vi "test_read-nmea-data2.vi"() -> ()   [LabVIEW 2019] (continued)
1.05,4*0A\n\t\n15:09:20.38\tF9P\t$GPGSV,3,1,09,02,54,318,23,04,19,044,21,05,36,246,28,06,65,046,30,1*66\n\t\n15:09:20.40\tF9P\t$GPGSV,3,2,09,09,45,075,25,12,24,278,29,17,34,153,23,19,53,156,23,1*68\n\t\n15:09:20.42\tF9P\t$GPGSV,3,3,09,25,12,308,,1*52\n\t\n15:09:20.44\tF9P\t$GPGSV,3,1,09,02,54,318,,04,19,044,15,05,36,246,18,06,65,046,22,6*67\n\t\n15:09:20.46\tF9P\t$GPGSV,3,2,09,09,45,075,18,12,24,278,17,17,34,153,,19,53,156,,6*6C\n\t\n15:09:20.48\tF9P\t$GPGSV,3,3,09,25,12,308,,6*55\n\t\n15:09:20.50\tF9P\t$GLGSV,2,1,08,69,13,031,,70,73,042,,71,50,204,32,72,03,209,,1*70\n\t\n15:09:20.52\tF9P\t$GLGSV,2,2,08,77,01,327,,84,21,121,13,85,70,063,25,86,35,329,,1*70\n\t\n15:09:20.54\tF9P\t$GLGSV,2,1,08,69,13,031,17,70,73,042,,71,50,204,23,72,03,209,,3*74\n\t\n15:09:20.56\tF9P\t$GLGSV,2,2,08,77,01,327,,84,21,121,17,85,70,063,20,86,35,329,,3*73\n\t\n15:09:20.58\tF9P\t$GAGSV,2,1,08,02,09,298,11,04,65,120,30,09,30,193,18,11,70,356,20,7*7A\n\t\n15:09:20.60\tF9P\t$GAGSV,2,2,08,12,41,101,18,19,27,046,08,25,10,250,,36,25,307,18,7*7D\n\t\n15:09:20.62\tF9P\t$GAGSV,2,1,08,02,09,298,,04,65,120,32,09,30,193,17,11,70,356,18,2*79\n\t\n15:09:20.64\tF9P\t$GAGSV,2,2,08,12,41,101,17,19,27,046,,25,10,250,,36,25,307,22,2*76\n\t\n15:09:20.66\tF9P\t$GBGSV,1,1,03,11,51,130,21,14,86,148,25,33,59,218,25,1*41\n\t\n15:09:20.68\tF9P\t$GBGSV,1,1,04,08,,,24,11,51,130,20,14,86,148,25,33,59,218,,3*4C\n\t\n15:09:20.70\tF9P\t$GNGLL,3723.60443,N,12656.90761,E,060922.00,A,A*77\n\t\n15:09:20.72\tF9P\t\t\n15:09:20.74\tF9P\t\t\n15:09:20.76\tF9P\t\t\n15:09:20.78\tF9P\t\t\n15:09:20.80\tF9P\t\t\n15:09:20.82\tF9P\t\t\n15:09:20.84\tF9P\t\t\n15:09:20.86\tF9P\t\t\n15:09:20.88\tF9P\t\t\n15:09:20.90\tF9P\t\t\n15:09:20.92\tF9P\t\t\n15:09:20.94\tF9P\t\t\n15:09:20.96\tF9P\t\t\n15:09:20.98\tF9P\t\t\n15:09:21.00\tF9P\t\t\n15:09:21.02\tF9P\t\t\n15:09:21.04\tF9P\t\t\n15:09:21.06\tF9P\t\t\n15:09:21.08\tF9P\t\t\n15:09:21.10\tF9P\t\t\n15:09:21.12\tF9P\t\t\n15:09:21.14\tF9P\t\t\n15:09:21.16\tF9P\t\t\n15:09:21.18\tF9P\t\t\n15:09:21.20\tF9P\t\t\n15:09:21.22\tF9P\t\t\n15:09:21.24\tF9P\t$GNRMC,060923.00,A,3723.60417,N,12656.90709,E,1.682,,250720,,,A,V*15\n\t\n15:09:21.26\tF9P\t$GNVTG,,T,,M,1.682,N,3.115,K,A*36\n\t\n15:09:21.28\tF9P\t$GNGGA,060923.00,3723.60417,N,12656.90709,E,1,12,0.73,58.2,M,18.5,M,,*78\n\t\n15:09:21.30\tF9P\t$GNGSA,A,3,12,06,19,05,17,09,04,02,,,,,1.28,0.73,1.05,1*0B\n\t\n15:09:21.32\tF9P\t$GNGSA,A,3,85,71,84,,,,,,,,,,1.28,0.73,1.05,2*0E\n\t\n15:09:21.34\tF9P\t$GNGSA,A,3,36,19,11,04,09,12,,,,,,,1.28,0.73,1.05,3*0B\n\t\n15:09:21.36\tF9P\t$GNGSA,A,3,14,11,33,,,,,,,,,,1.28,0.73,1.05,4*0A\n\t\n15:09:21.38\tF9P\t$GPGSV,3,1,09,02,54,318,24,04,19,044,20,05,36,246,28,06,65,046,30,1*60\n\t\n15:09:21.40\tF9P\t$GPGSV,3,2,09,09,45,075,25,12,24,278,29,17,34,153,23,19,53,156,24,1*6F\n\t\n15:09:21.42\tF9P\t$GPGSV,3,3,09,25,12,308,,1*52\n\t\n15:09:21.44\tF9P\t$GPGSV,3,1,09,02,54,318,,04,19,044,14,05,36,246,18,06,65,046,24,6*60\n\t\n15:09:21.46\tF9P\t$GPGSV,3,2,09,09,45,075,18,12,24,278,18,17,34,153,,19,53,156,,6*63\n\t\n15:09:21.48\tF9P\t$GPGSV,3,3,09,25,12,308,,6*55\n\t\n15:09:21.50\tF9P\t$GLGSV,2,1,08,69,13,031,,70,73,042,,71,50,204,28,72,03,209,,1*7B\n\t\n15:09:21.52\tF9P\t$GLGSV,2,2,08,77,01,327,,84,21,121,11,85,70,063,30,86,35,329,,1*76\n\t\n15:09:21.54\tF9P\t$GLGSV,2,1,08,69,13,031,19,70,73,042,,71,50,204,22,72,03,209,,3*7B\n\t\n15:09:21.56\tF9P\t$GLGSV,2,2,08,77,01,327,,84,21,121,19,85,70,063,20,86,35,329,,3*7D\n\t\n15:09:21.58\tF9P\t$GAGSV,2,1,08,02,09,298,15,04,65,120,21,09,30,193,17,11,70,356,20,7*71\n\t\n15:09:21.60\tF9P\t$GAGSV,2,2,08,12,41,101,20,19,27,046,17,25,10,250,,36,25,307,20,7*73\n\t\n15:09:21.62\tF9P\t$GAGSV,2,1,08,02,09,298,,04,65,120,27,09,30,193,17,11,70,356,18,2*7D\n\t\n15:09:21.64\tF9P\t$GAGSV,2,2,08,12,41,101,16,19,27,046,,25,10,250,,36,25,307,19,2*7F\n\t\n15:09:21.66\tF9P\t$GBGSV,1,1,03,11,51,130,22,14,86,148,25,33,59,218,26,1*41\n\t\n15:09:21.68\tF9P\t$GBGSV,1,1,04,08,,,25,11,51,130,21,14,86,148,24,33,59,218,,3*4D\n\t\n15:09:21.70\tF9P\t$GNGLL,3723.60417,N,12656.90709,E,060923.00,A,A*79\n\t\n15:09:21.72\tF9P\t\t\n15:09:21.74\tF9P\t\t\n15:09:21.76\tF9P\t\t\n15:09:21.78\tF9P\t\t\n15:09:21.80\tF9P\t\t\n15:09:21.82\tF9P\t\t\n15:09:21.84\tF9P\t\t\n15:09:21.86\tF9P\t\t\n15:09:21.88\tF9P\t\t\n15:09:21.90\tF9P\t\t\n15:09:21.92\tF9P\t\t\n15:09:21.94\tF9P\t\t\n15:09:21.96\tF9P\t\t\n15:09:21.98\tF9P\t\t\n15:09:22.00\tF9P\t\t\n15:09:22.02\tF9P\t\t\n15:09:22.04\tF9P\t\t\n15:09:22.06\tF9P\t\t\n15:09:22.08\tF9P\t\t\n15:09:22.10\tF9P\t\t\n15:09:22.12\tF9P\t\t\n15:09:22.14\tF9P\t\t\n15:09:22.16\tF9P\t\t\n15:09:22.18\tF9P\t\t\n15:09:22.20\tF9P\t\t\n15:09:22.22\tF9P\t\t\n15:09:22.24\tF9P\t$GNRMC,060924.00,A,3723.60402,N,12656.90651,E,1.519,,250720,,,A,V*1B\n\t\n15:09:22.26\tF9P\t$GNVTG,,T,,M,1.519,N,2.813,K,A*39\n\t\n15:09:22.28\tF9P\t$GNGGA,060924.00,3723.60402,N,12656.90651,E,1,12,0.73,58.0,M,18.5,M,,*75\n\t\n15:09:22.30\tF9P\t$GNGSA,A,3,12,06,19,05,17,09,04,02,,,,,1.28,0.73,1.05,1*0B\n\t\n15:09:22.32\tF9P\t$GNGSA,A,3,85,71,84,,,,,,,,,,1.28,0.73,1.05,2*0E\n\t\n15:09:22.34\tF9P\t$GNGSA,A,3,36,19,11,04,09,12,,,,,,,1.28,0.73,1.05,3*0B\n\t\n15:09:22.36\tF9P\t$GNGSA,A,3,14,11,33,,,,,,,,,,1.28,0.73,1.05,4*0A\n\t\n15:09:22.38\tF9P\t$GPGSV,3,1,09,02,54,318,23,04,19,044,19,05,36,246,28,06,65,046,28,1*64\n\t\n15:09:22.40\tF9P\t$GPGSV,3,2,09,09,45,075,25,12,24,278,29,17,34,153,25,19,53,156,24,1*69\n\t\n15:09:22.43\tF9P\t$GPGSV,3,3,09,25,12,307,,1*5D\n\t\n15:09:22.45\tF9P\t$GPGSV,3,1,09,02,54,318,,04,19,044,13,05,36,246,20,06,65,046,23,6*6B\n\t\n15:09:22.47\tF9P\t$GPGSV,3,2,09,09,45,075,18,12,24,278,16,17,34,153,,19,53,156,,6*6D\n\t\n15:09:22.49\tF9P\t$GPGSV,3,3,09,25,12,307,,6*5A\n\t\n15:09:22.51\tF9P\t$GLGSV,2,1,08,69,13,031,,70,73,042,,71,50,204,28,72,03,209,,1*7B\n\t\n15:09:22.53\tF9P\t$GLGSV,2,2,08,77,01,327,,84,21,121,10,85,70,063,25,86,35,329,,1*73\n\t\n15:09:22.55\tF9P\t$GLGSV,2,1,08,69,13,031,20,70,73,042,,71,50,204,22,72,03,209,,3*71\n\t\n15:09:22.57\tF9P\t$GLGSV,2,2,08,77,01,327,,84,21,121,18,85,70,063,21,86,35,329,,3*7D\n\t\n15:09:22.59\tF9P\t$GAGSV,2,1,08,02,09,298,23,04,65,120,21,09,30,193,16,11,70,356,19,7*7F\n\t\n15:09:22.61\tF9P\t$GAGSV,2,2,08,12,41,101,19,19,27,046,10,25,10,250,,36,25,307,21,7*7F\n\t\n15:09:22.63\tF9P\t$GAGSV,2,1,08,02,09,298,,04,65,120,33,09,30,193,14,11,70,356,16,2*75\n\t\n15:09:22.65\tF9P\t$GAGSV,2,2,08,12,41,101,13,19,27,046,,25,10,250,,36,25,307,18,2*7B\n\t\n15:09:22.67\tF9P\t$GBGSV,1,1,03,11,51,130,22,14,86,148,26,33,59,218,25,1*41\n\t\n15:09:22.69\tF9P\t$GBGSV,1,1,04,08,,,24,11,51,130,21,14,86,148,25,33,59,218,,3*4D\n\t\n15:09:22.71\tF9P\t$GNGLL,3723.60402,N,12656.90651,E,060924.00,A,A*76\n\t\n15:09:22.73\tF9P\t\t\n15:09:22.75\tF9P\t\t\n15:09:22.77\tF9P\t\t\n15:09:22.79\tF9P\t\t\n15:09:22.81\tF9P\t\t\n15:09:22.83\tF9P\t\t\n15:09:22.85\tF9P\t\t\n15:09:22.87\tF9P\t\t\n15:09:22.89\tF9P\t\t\n15:09:22.91\tF9P\t\t\n15:09:22.93\tF9P\t\t\n15:09:22.95\tF9P\t\t\n15:09:22.97\tF9P\t\t\n15:09:22.99\tF9P\t\t\n15:09:23.01\tF9P\t\t\n15:09:23.03\tF9P\t\t\n15:09:23.05\tF9P\t\t\n15:09:23.07\tF9P\t\t\n15:09:23.09\tF9P\t\t\n15:09:23.11\tF9P\t\t\n15:09:23.13\tF9P\t\t\n15:09:23.15\tF9P\t\t\n15:09:23.17\tF9P\t\t\n15:09:23.19\tF9P\t\t\n15:09:23.21\tF9P\t\t\n15:09:23.23\tF9P\t\t\n15:09:23.25\tF9P\t$GNRMC,060925.00,A,3723.60390,N,12656.90580,E,1.871,,250720,,,A,V*1A\n\t\n15:09:23.27\tF9P\t$GNVTG,,T,,M,1.871,N,3.465,K,A*36\n\t\n15:09:23.29\tF9P\t$GNGGA,060925.00,3723.60390,N,12656.90580,E,1,12,0.76,57.8,M,18.5,M,,*75\n\t\n15:09:23.32\tF9P\t$GNGSA,A,3,12,06,19,05,17,09,04,02,,,,,1.33,0.76,1.09,1*08\n\t\n15:09:23.34\tF9P\t$GNGSA,A,3,85,71,84,,,,,,,,,,1.33,0.76,1.09,2*0D\n\t\n15:09:23.36\tF9P\t$GNGSA,A,3,36,19,11,04,09,12,,,,,,,1.33,0.76,1.09,3*08\n\t\n15:09:23.38\tF9P\t$GNGSA,A,3,14,11,33,,,,,,,,,,1.33,0.76,1.09,4*09\n\t\n15:09:23.40\tF9P\t$GPGSV,3,1,09,02,54,318,24,04,19,044,20,05,36,246,29,06,65,046,28,1*68\n\t\n15:09:23.42\tF9P\t$GPGSV,3,2,09,09,45,075,24,12,24,278,28,17,34,153,23,19,53,156,23,1*68\n\t\n15:09:23.44\tF9P\t$GPGSV,3,3,09,25,12,307,26,1*59\n\t\n15:09:23.46\tF9P\t$GPGSV,3,1,09,02,54,318,,04,19,044,13,05,36,246,20,06,65,046,20,6*68\n\t\n15:09:23.48\tF9P\t$GPGSV,3,2,09,09,45,075,19,12,24,278,16,17,34,153,,19,53,156,,6*6C\n\t\n15:09:23.50\tF9P\t$GPGSV,3,3,09,25,12,307,,6*5A\n\t\n15:09:23.52\tF9P\t$GLGSV,2,1,08,69,13,031,,70,73,042,,71,50,204,27,72,03,209,,1*74\n\t\n15:09:23.54\tF9P\t$GLGSV,2,2,08,77,01,327,,84,21,121,07,85,70,063,25,86,35,329,,1*75\n\t\n15:09:23.56\tF9P\t$GLGSV,2,1,08,69,13,031,22,70,73,042,,71,50,204,23,72,03,209,,3*72\n\t\n15:09:23.58\tF9P\t$GLGSV,2,2,08,77,01,327,,84,21,121,18,85,70,063,22,86,35,329,,3*7E\n\t\n15:09:23.60\tF9P\t$GAGSV,2,1,08,02,09,298,22,04,65,120,23,09,30,193,16,11,70,356,20,7*76\n\t\n15:09:23.62\tF9P\t$GAGSV,2,2,08,12,41,101,19,19,27,046,13,25,10,250,,36,25,307,22,7*7F\n\t\n15:09:23.64\tF9P\t$GAGSV,2,1,08,02,09,298,,04,65,120,32,09,30,193,13,11,70,356,19,2*7C\n\t\n15:09:23.66\tF9P\t$GAGSV,2,2,08,12,41,101,,19,27,046,,25,10,250,,36,25,307,16,2*77\n\t\n15:09:23.68\tF9P\t$GBGSV,1,1,03,11,51,130,22,14,86,148,26,33,59,218,30,1*45\n\t\n15:09:23.70\tF9P\t$GBGSV,1,1,04,08,,,23,11,51,130,23,14,86,148,26,33,59,218,,3*4B\n\t\n15:09:23.72\tF9P\t$GNGLL,3723.60390,N,12656.90580,E,060925.00,A,A*74\n\t\n15:09:23.74\tF9P\t\t\n15:09:23.76\tF9P\t\t\n15:09:23.78\tF9P\t\t\n15:09:23.80\tF9P\t\t\n15:09:23.82\tF9P\t\t\n15:09:23.84\tF9P\t\t\n15:09:23.86\tF9P\t\t\n15:09:23.88\tF9P\t\t\n15:09:23.90\tF9P\t\t\n15:09:23.92\tF9P\t\t\n15:09:23.94\tF9P\t\t\n15:09:23.96\tF9P\t\t\n15:09:23.98\tF9P\t\t\n15:09:24.00\tF9P\t\t\n15:09:24.02\tF9P\t\t\n15:09:24.04\tF9P\t\t\n15:09:24.06\tF9P\t\t\n15:09:24.08\tF9P\t\t\n15:09:24.10\tF9P\t\t\n15:09:24.12\tF9P\t\t\n15:09:24.14\tF9P\t\t\n15:09:24.16\tF9P\t\t\n15:09:24.18\tF9P\t\t\n15:09:24.20\tF9P\t\t\n15:09:24.22\tF9P\t\t\n15:09:24.24\tF9P\t$GNRMC,060926.00,A,3723.60386,N,12656.90524,E,1.422,,250720,,,A,V*1A\n\t\n15:09:24.26\tF9P\t$GNVTG,,T,,M,1.422,N,2.634,K,A*3B\n\t\n15:09:24.28\tF9P\t$GNGGA,060926.00,3723.60386,N,12656.90524,E,1,12,0.66,58.2,M,18.5,M,,*7B\n\t\n15:09:24.30\tF9P\t$GNGSA,A,3,12,06,19,05,17,09,04,02,,,,,1.21,0.66,1.01,1*02\n\t\n15:09:24.32\tF9P\t$GNGSA,A,3,85,71,84,,,,,,,,,,1.21,0.66,1.01,2*07\n\t\n15:09:24.34\tF9P\t$GNGSA,A,3,36,19,11,04,09,12,,,,,,,1.21,0.66,1.01,3*02\n\t\n15:09:24.36\tF9P\t$GNGSA,A,3,14,11,33,,,,,,,,,,1.21,0.66,1.01,4*03\n\t\n15:09:24.38\tF9P\t$GPGSV,3,1,09,02,54,318,24,04,19,044,20,05,36,246,27,06,65,046,29,1*67\n\t\n15:09:24.40\tF9P\t$GPGSV,3,2,09,09,45,075,25,12,24,278,27,17,34,153,23,19,53,156,23,1*66\n\t\n15:09:24.42\tF9P\t$GPGSV,3,3,09,25,12,307,31,1*5F\n\t\n15:09:24.44\tF9P\t$GPGSV,3,1,09,02,54,318,,04,19,044,14,05,36,246,20,06,65,046,18,6*64\n\t\n15:09:24.46\tF9P\t$GPGSV,3,2,09,09,45,075,20,12,24,278,15,17,34,153,,19,53,156,,6*65\n\t\n15:09:24.48\tF9P\t$GPGSV,3,3,09,25,12,307,,6*5A\n\t\n15:09:24.50\tF9P\t$GLGSV,2,1,08,69,13,031,,70,73,042,,71,50,204,25,72,03,209,,1*76\n\t\n15:09:24.52\tF9P\t$GLGSV,2,2,08,77,01,327,,84,21,121,13,85,70,063,26,86,35,329,,1*73\n\t\n15:09:24.54\tF9P\t$GLGSV,2,1,08,69,13,031,21,70,73,042,,71,50,204,22,72,03,209,,3*70\n\t\n15:09:24.56\tF9P\t$GLGSV,2,2,08,77,01,327,,84,21,121,16,85,70,063,22,86,35,329,,3*70\n\t\n15:09:24.58\tF9P\t$GAGSV,2,1,08,02,09,298,26,04,65,120,26,09,30,193,15,11,70,356,20,7*74\n\t\n15:09:24.60\tF9P\t$GAGSV,2,2,08,12,41,101,19,19,27,046,13,25,10,250,,36,25,307,34,7*78\n\t\n15:09:24.62\tF9P\t$GAGSV,2,1,08,02,09,298,,04,65,120,35,09,30,193,11,11,70,356,19,2*79\n\t\n15:09:24.64\tF9P\t$GAGSV,2,2,08,12,41,101,,19,27,046,,25,10,250,,36,25,307,,2*70\n\t\n15:09:24.66\tF9P\t$GBGSV,1,1,03,11,51,130,23,14,86,148,26,33,59,218,24,1*41\n\t\n15:09:24.68\tF9P\t$GBGSV,1,1,04,08,,,23,11,51,130,23,14,86,148,26,33,59,218,,3*4B\n\t\n15:09:24.70\tF9P\t$GNGLL,3723.60386,N,12656.90524,E,060926.00,A,A*7E\n\t\n15:09:24.72\tF9P\t\t\n15:09:24.74\tF9P\t\t\n15:09:24.76\tF9P\t\t\n15:09:24.78\tF9P\t\t\n15:09:24.80\tF9P\t\t\n15:09:24.82\tF9P\t\t\n15:09:24.84\tF9P\t\t\n15:09:24.86\tF9P\t\t\n15:09:24.88\tF9P\t\t\n15:09:24.90\tF9P\t\t\n15:09:24.92\tF9P\t\t\n15:09:24.94\tF9P\t\t\n15:09:24.96\tF9P\t\t\n15:09:24.98\tF9P\t\t\n15:09:25.00\tF9P\t\t\n15:09:25.02\tF9P\t\t\n15:09:25.04\tF9P\t\t\n15:09:25.06\tF9P\t\t\n15:09:25.08\tF9P\t\t\n15:09:25.10\tF9P\t\t\n15:09:25.12\tF9P\t\t\n15:09:25.14\tF9P\t\t\n15:09:25.16\tF9P\t\t\n15:09:25.18\tF9P\t\t\n15:09:25.20\tF9P\t\t\n15:09:25.22\tF9P\t\t\n15:09:25.24\tF9P\t$GNRMC,060927.00,A,3723.60381,N,12656.90446,E,2.414,257.19,250720,,,A,V*09\n\t\n15:09:25.26\tF9P\t$GNVTG,257.19,T,,M,2.414,N,4.470,K,A*2F\n\t\n15:09:25.28\tF9P\t$GNGGA,060927.00,3723.60381,N,12656.90446,E,1,12,0.66,57.8,M,18.5,M,,*7D\n\t\n15:09:25.30\tF9P\t$GNGSA,A,3,12,06,19,05,17,09,04,02,,,,,1.21,0.66,1.01,1*02\n\t\n15:09:25.32\tF9P\t$GNGSA,A,3,85,71,84,,,,,,,,,,1.21,0.66,1.01,2*07\n\t\n15:09:25.34\tF9P\t$GNGSA,A,3,36,19,11,04,09,12,,,,,,,1.21,0.66,1.01,3*02\n\t\n15:09:25.36\tF9P\t$GNGSA,A,3,14,11,33,,,,,,,,,,1.21,0.66,1.01,4*03\n\t\n15:09:25.38\tF9P\t$GPGSV,3,1,09,02,54,318,24,04,19,044,19,05,36,246,27,06,65,046,34,1*61\n\t\n15:09:25.40\tF9P\t$GPGSV,3,2,09,09,45,075,27,12,24,278,26,17,34,153,21,19,53,156,22,1*66\n\t\n15:09:25.42\tF9P\t$GPGSV,3,3,09,25,12,307,31,1*5F\n\t\n15:09:25.44\tF9P\t$GPGSV,3,1,09,02,54,318,,04,19,044,13,05,36,246,21,06,65,046,20,6*69\n\t\n15:09:25.46\tF9P\t$GPGSV,3,2,09,09,45,075,19,12,24,278,16,17,34,153,,19,53,156,,6*6C\n\t\n15:09:25.48\tF9P\t$GPGSV,3,3,09,25,12,307,,6*5A\n\t\n15:09:25.50\tF9P\t$GLGSV,2,1,08,69,13,031,,70,73,042,,71,50,204,25,72,03,209,,1*76\n\t\n15:09:25.52\tF9P\t$GLGSV,2,2,08,77,01,327,,84,21,121,13,85,70,063,25,86,35,329,,1*70\n\t\n15:09:25.54\tF9P\t$GLGSV,2,1,08,69,13,031,21,70,73,042,,71,50,204,21,72,03,209,,3*73\n\t\n15:09:25.56\tF9P\t$GLGSV,2,2,08,77,01,327,,84,21,121,15,85,70,063,21,86,35,329,,3*70\n\t\n15:09:25.58\tF9P\t$GAGSV,2,1,08,02,09,298,25,04,65,120,24,09,30,193,15,11,70,356,19,7*7F\n\t\n15:09:25.60\tF9P\t$GAGSV,2,2,08,12,41,101,18,19,27,046,14,25,10,250,,36,25,307,32,7*78\n\t\n15:09:25.62\tF9P\t$GAGSV,2,1,08,02,09,298,,04,65,120,26,09,30,193,,11,70,356,20,2*71\n\t\n15:09:25.64\tF9P\t$GAGSV,2,2,08,12,41,101,,19,27,046,,25,10,250,,36,25,307,,2*70\n\t\n15:09:25.66\tF9P\t$GBGSV,1,1,03,11,51,130,22,14,86,148,25,33,59,218,29,1*4E\n\t\n15:09:25.68\tF9P\t$GBGSV,1,1,04,08,,,22,11,51,130,23,14,86,148,30,33,59,218,,3*4D\n\t\n15:09:25.70\tF9P\t$GNGLL,3723.60381,N,12656.90446,E,060927.00,A,A*7D\n\t\n15:09:25.72\tF9P\t\t\n15:09:25.74\tF9P\t\t\n15:09:25.76\tF9P\t\t\n15:09:25.78\tF9P\t\t\n15:09:25.80\tF9P\t\t\n15:09:25.82\tF9P\t\t\n15:09:25.84\tF9P\t\t\n15:09:25.86\tF9P\t\t\n15:09:25.88\tF9P\t\t\n15:09:25.90\tF9P\t\t\n15:09:25.92\tF9P\t\t\n15:09:25.94\tF9P\t\t\n15:09:25.96\tF9P\t\t\n15:09:25.98\tF9P\t\t\n15:09:26.00\tF9P\t\t\n15:09:26.02\tF9P\t\t\n15:09:26.04\tF9P\t\t\n15:09:26.06\tF9P\t\t\n15:09:26.08\tF9P\t\t\n15:09:26.10\tF9P\t\t\n15:09:26.12\tF9P\t\t\n15:09:26.14\tF9P\t\t\n15:09:26.16\tF9P\t\t\n15:09:26.18\tF9P\t\t\n15:09:26.20\tF9P\t\t\n15:09:26.22\tF9P\t\t\n15:09:26.24\tF9P\t\t\n15:09:26.26\tF9P\t$GNRMC,060928.00,A,3723.60370,N,12656.90424,E,0.679,,250720,,,A,V*11\n\t\n15:09:26.28\tF9P\t$GNVTG,,T,,M,0.679,N,1.257,K,A*34\n\t\n15:09:26.30\tF9P\t$GNGGA,060928.00,3723.60370,N,12656.90424,E,1,12,0.64,57.0,M,18.5,M,,*72\n\t\n15:09:26.32\tF9P\t$GNGSA,A,3,12,06,19,05,17,09,04,02,,,,,1.19,0.64,1.00,1*0A\n\t\n15:09:26.34\tF9P\t$GNGSA,A,3,85,71,84,,,,,,,,,,1.19,0.64,1.00,2*0F\n\t\n15:09:26.36\tF9P\t$GNGSA,A,3,36,19,11,04,09,12,,,,,,,1.19,0.64,1.00,3*0A\n\t\n15:09:26.38\tF9P\t$GNGSA,A,3,14,11,33,,,,,,,,,,1.19,0.64,1.00,4*0B\n\t\n15:09:26.40\tF9P\t$GPGSV,3,1,09,02,54,318,31,04,19,044,18,05,36,246,26,06,65,046,30,1*61\n\t\n15:09:26.42\tF9P\t$GPGSV,3,2,09,09,45,075,33,12,24,278,26,17,34,153,29,19,53,156,22,1*6B\n\t\n15:09:26.44\tF9P\t$GPGSV,3,3,09,25,12,307,35,1*5B\n\t\n15:09:26.46\tF9P\t$GPGSV,3,1,09,02,54,318,,04,19,044,12,05,36,246,20,06,65,046,21,6*68\n\t\n15:09:26.48\tF9P\t$GPGSV,3,2,09,09,45,075,18,12,24,278,15,17,34,153,,19,53,156,,6*6E\n\t\n15:09:26.50\tF9P\t$GPGSV,3,3,09,25,12,307,,6*5A\n\t\n15:09:26.52\tF9P\t$GLGSV,2,1,08,69,13,031,,70,73,042,,71,50,204,30,72,03,209,,1*72\n\t\n15:09:26.54\tF9P\t$GLGSV,2,2,08,77,01,327,,84,21,121,09,85,70,063,26,86,35,329,,1*78\n\t\n15:09:26.56\tF9P\t$GLGSV,2,1,08,69,13,031,20,70,73,042,,71,50,204,20,72,03,209,,3*73\n\t\n15:09:26.58\tF9P\t$GLGSV,2,2,08,77,01,327,,84,21,121,18,85,70,063,20,86,35,329,,3*7C\n\t\n15:09:26.60\tF9P\t$GAGSV,2,1,08,02,09,298,25,04,65,120,24,09,30,193,15,11,70,356,19,7*7F\n\t\n15:09:26.62\tF9P\t$GAGSV,2,2,08,12,41,101,17,19,27,046,13,25,10,250,,36,25,307,27,7*74\n\t\n15:09:26.64\tF9P\t$GAGSV,2,1,08,02,09,298,,04,65,120,27,09,30,193,,11,70,356,19,2*7A\n\t\n15:09:26.66\tF9P\t$GAGSV,2,2,08,12,41,101,,19,27,046,,25,10,250,,36,25,307,30,2*73\n\t\n15:09:26.68\tF9P\t$GBGSV,1,1,03,11,51,130,22,14,86,148,25,33,59,218,22,1*45\n\t\n15:09:26.70\tF9P\t$GBGSV,1,1,04,08,,,21,11,51,130,23,14,86,148,28,33,59,218,,3*47\n\t\n15:09:26.72\tF9P\t$GNGLL,3723.60370,N,12656.90424,E,060928.00,A,A*78\n\t\n15:09:26.74\tF9P\t\t\n15:09:26.76\tF9P\t\t\n15:09:26.78\tF9P\t\t\n15:09:26.80\tF9P\t\t\n15:09:26.82\tF9P\t\t\n15:09:26.84\tF9P\t\t\n15:09:26.86\tF9P\t\t\n15:09:26.88\tF9P\t\t\n15:09:26.90\tF9P\t\t\n15:09:26.92\tF9P\t\t\n15:09:26.94\tF9P\t\t\n15:09:26.96\tF9P\t\t\n15:09:26.98\tF9P\t\t\n15:09:27.00\tF9P\t\t\n15:09:27.02\tF9P\t\t\n15:09:27.04\tF9P\t\t\n15:09:27.06\tF9P\t\t\n15:09:27.08\tF9P\t\t\n15:09:27.10\tF9P\t\t\n15:09:27.12\tF9P\t\t\n15:09:27.14\tF9P\t\t\n15:09:27.16\tF9P\t\t\n15:09:27.18\tF9P\t\t\n15:09:27.20\tF9P\t\t\n15:09:27.22\tF9P\t\t\n15:09:27.24\tF9P\t$GNRMC,060929.00,A,3723.60349,N,12656.90376,E,1.544,,250720,,,A,V*16\n\t\n15:09:27.26\tF9P\t$GNVTG,,T,,M,1.544,N,2.860,K,A*35\n\t\n15:09:27.28\tF9P\t$GNGGA,060929.00,3723.60349,N,12656.90376,E,1,12,0.64,57.5,M,18.5,M,,*7C\n\t\n15:09:27.30\tF9P\t$GNGSA,A,3,12,06,19,05,17,09,04,02,,,,,1.19,0.64,1.00,1*0A\n\t\n15:09:27.32\tF9P\t$GNGSA,A,3,85,71,84,,,,,,,,,,1.19,0.64,1.00,2*0F\n\t\n15:09:27.34\tF9P\t$GNGSA,A,3,36,19,11,04,09,12,,,,,,,1.19,0.64,1.00,3*0A\n\t\n15:09:27.36\tF9P\t$GNGSA,A,3,14,11,33,,,,,,,,,,1.19,0.64,1.00,4*0B\n\t\n15:09:27.38\tF9P\t$GPGSV,3,1,09,02,54,318,29,04,19,044,21,05,36,246,25,06,65,046,30,1*61\n\t\n15:09:27.40\tF9P\t$GPGSV,3,2,09,09,45,075,28,12,24,278,26,17,34,153,23,19,53,156,24,1*6D\n\t\n15:09:27.42\tF9P\t$GPGSV,3,3,09,25,12,307,27,1*58\n\t\n15:09:27.44\tF9P\t$GPGSV,3,1,09,02,54,318,,04,19,044,14,05,36,246,19,06,65,046,21,6*64\n\t\n15:09:27.46\tF9P\t$GPGSV,3,2,09,09,45,075,20,12,24,278,16,17,34,153,,19,53,156,,6*66\n\t\n15:09:27.48\tF9P\t$GPGSV,3,3,09,25,12,307,,6*5A\n\t\n15:09:27.50\tF9P\t$GLGSV,2,1,08,69,13,031,,70,73,042,,71,50,204,26,72,03,209,,1*75\n\t\n15:09:27.52\tF9P\t$GLGSV,2,2,08,77,01,327,,84,21,121,08,85,70,063,25,86,35,329,,1*7A\n\t\n15:09:27.54\tF9P\t$GLGSV,2,1,08,69,13,031,19,70,73,042,,71,50,204,22,72,03,209,,3*7B\n\t\n15:09:27.56\tF9P\t$GLGSV,2,2,08,77,01,327,,84,21,121,18,85,70,063,20,86,35,329,,3*7C\n\t\n15:09:27.58\tF9P\t$GAGSV,2,1,08,02,09,298,23,04,65,120,25,09,30,193,15,11,70,356,19,7*78\n\t\n15:09:27.60\tF9P\t$GAGSV,2,2,08,12,41,101,19,19,27,046,14,25,10,250,,36,25,307,27,7*7D\n\t\n15:09:27.62\tF9P\t$GAGSV,2,1,08,02,09,298,,04,65,120,25,09,30,193,,11,70,356,18,2*79\n\t\n15:09:27.64\tF9P\t$GAGSV,2,2,08,12,41,101,,19,27,046,,25,10,250,,36,25,307,23,2*71\n\t\n15:09:27.66\tF9P\t$GBGSV,1,1,03,11,51,130,20,14,86,148,26,33,59,218,29,1*4F\n\t\n15:09:27.68\tF9P\t$GBGSV,1,1,04,08,,,22,11,51,130,23,14,86,148,28,33,59,218,,3*44\n\t\n15:09:27.70\tF9P\t$GNGLL,3723.60349,N,12656.90376,E,060929.00,A,A*73\n\t\n15:09:27.72\tF9P\t\t\n15:09:27.74\tF9P\t\t\n15:09:27.76\tF9P\t\t\n15:09:27.78\tF9P\t\t\n15:09:27.80\tF9P\t\t\n15:09:27.82\tF9P\t\t\n15:09:27.84\tF9P\t\t\n15:09:27.86\tF9P\t\t\n15:09:27.88\tF9P\t\t\n15:09:27.90\tF9P\t\t\n15:09:27.92\tF9P\t\t\n15:09:27.94\tF9P\t\t\n15:09:27.96\tF9P\t\t\n15:09:27.98\tF9P\t\t\n15:09:28.00\tF9P\t\t\n15:09:28.02\tF9P\t\t\n15:09:28.04\tF9P\t\t\n15:09:28.06\tF9P\t\t\n15:09:28.08\tF9P\t\t\n15:09:28.10\tF9P\t\t\n15:09:28.12\tF9P\t\t\n15:09:28.14\tF9P\t\t\n15:09:28.16\tF9P\t\t\n15:09:28.18\tF9P\t\t\n15:09:28.20\tF9P\t\t\n15:09:28.22\tF9P\t\t\n15:09:28.24\tF9P\t\t\n15:09:28.26\t
